vi "Component.Tabulator_Init.vi"(8 "Error In":errorcluster, 10 "WebView2 Control in":refnum<k24>(container), 11 "object in":refnum<class "Component.Tabulator.lvclass">) -> (0 "Error Out":errorcluster, 3 "object out":refnum<class "Component.Tabulator.lvclass">)   [LabVIEW 2020, in "Component.Tabulator.lvclass"]
uses:
  Component.Tabulator.lvclass
  <vilib>/sklein/WebView2/Webview2 Lib/WebView2 Control Object/WebView2 Control.lvclass
  Component.Tabulator.lvclass/Component.Tabulator.ctl
  Component_class/Component.lvclass
  <vilib>/sklein/WebView2/Libs/Microsoft.Web.WebView2.WinForms.dll
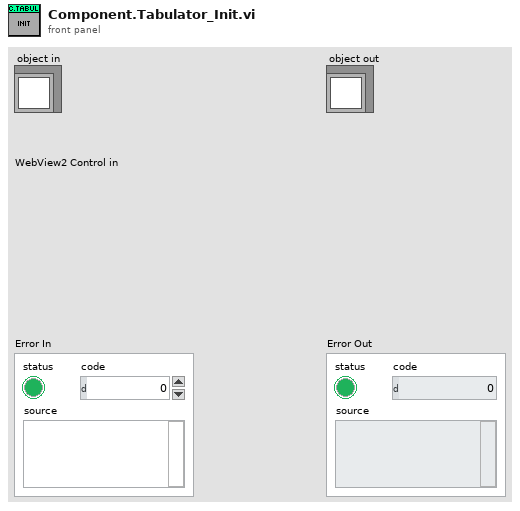
[diagram p1: front panel]
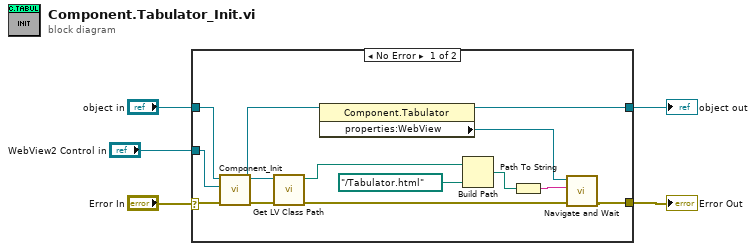
[diagram p0: block diagram]
diagram:
  n1 = case shown="No Error" "Error In" {
    selector: "Error In" -> [w18 w20]
    tunnel: [w10 w20] -> w4
    tunnel: "WebView2 Control in" -> [w14 _]
    tunnel: [w12 w19] -> w2
    tunnel: "object in" -> [w11 w19]
    frame No Error {
      n2 = call "Component_Init.vi"("Error In"=w18, "WebView2"=w14, "object in"=w11) -> ("Error Out"=w15:errorcluster, "object out"=w13:refnum<class "Component.Tabulator.lvclass">)  [unwired: 7 in]
      n3 = call <vilib>:"Get LV Class Path.vi"("error in (no error)"=w15, "object"=w13) -> ("error out"=w9:errorcluster, "class path"=w17:path)  [unwired: 8 in]
      n4 = property class="Component.Tabulator"(reference=w13) -> (reference out=w12:refnum<class "Component.Tabulator.lvclass">, "properties:WebView"=w8:refnum<class "WebView2 Control.lvclass">)  [unwired: 1 in, 1 out]
      n5 = Build Path(base path=w17, name or relative path=path "../Tabulator.html") -> (appended path=w7:path)
      n6 = Path To String(path=w7) -> (string=w6:string)
      n7 = call <vilib>:"Navigate and Wait.vi"("error in (no error)"=w9, "Source"=w6, "WebView2 Control in"=w8) -> ("error out"=w10:errorcluster)  [unwired: 6 in, 2 out]
    }
    frame Error {
    }
  }
  "object out" <- w2
  "Error Out" <- w4
